vi "main_original.vi"() -> ()   [LabVIEW 2010]
uses:
  common_typedefs/channels_cluster.ctl
  common_typedefs/clock_parameters_cluster.ctl
  scan_specification_cluster.ctl
  common_typedefs/DAC_voltage_cluster.ctl
  derived_values_cluster.ctl
  counter_cluster.ctl
  integration_cluster.ctl
  common_typedefs/DAC_values_cluster.ctl
  common_typedefs/DAC_channel_enable_cluster.ctl
  <vilib>/Platform/TimedLoop/XDataNode/XDataNode.xnode
  <vilib>/Platform/TimedLoop/XDataNode/timing_clust.ctl
  <vilib>/Platform/TimedLoop/XDataNode/nitl_modes.ctl
  <vilib>/Platform/TimedLoop/XDataNode/wakeup.ctl
  <vilib>/eio/EIONode/EIONode.xnode
  <vilib>/rvi/eio/nirviEIOImplementation/nirviEIOImplementation.xnode
  <vilib>/rvi/eio/common/nirviEmuClasses.ctl
  <vilib>/rvi/eio/common/nirviEmuTemplateMethod_noerrors.vi
  <vilib>/Platform/TimedLoop/XDataNode/XDNodeRunTimeDep.lvlib
panel:
  in  "sync minimum high":i16=1000
  out "PIXEL COUNTER":u64(graph)
  out "Loop time":u32=100
  out "line counter":u16(graph)
  out "finished?":bool
  in  "transfer extra-waitlines?":bool
  out "transferred extra waitlines":u32
  out "no of correct transferred z tuples":u32
  out "z-points transfer corrupt?":bool
  out "transferred z/intensity tuples":u32
  in  "transfer z-points?":bool
  in  "invert channels":bool[](array[boolean])=[FALSE, FALSE]
  in  "enable fly-back reversion?":bool=TRUE
  out "pixels acquired":u64
  out "counter cluster out":T1
  out "derived values":T2
  out "acquire?":bool
  in  "ADC clock phase":u8=2
  out "DAC voltages":T3 {"ch6" max=4095 step=1; "ch5" max=4095 step=1; "ch4" max=4095 step=1; "ch3" max=4095 step=1; "ch2" max=4095 step=1; "ch1" max=4095 step=1; "ch0" max=4095 step=1}
  in  "scan specification":T4={"x amplitude"=1000, "x resolution (pixels)"=100, "x offset fly-forward (iterations)"=0, "x offset fly-back (iterations)"=0, "y resolution (nr. of lines)"=200, "y step size"=5, "iterations per pixel"=5, "number of frames"=-1, "y offset (pixels)"=0, "number of y-brake lines  (before y-fly-back)"=2, "number y-brake lines (after y-fly-back)"=2, "number of y-fly-back steps"=2, "lines per z step"=5, "number of z/intensity tuples"=200, "number of repetitions (volumes or planes)"=500, "z step size derived"=0, "choose the beginning of z scan"=FALSE, "number of frames (settings)"=0, "FPGA trajectory?"=FALSE}
  out "clock 1 state":bool
  out "clock 2 state":bool
  out "clock 3 state":bool
  in  "clock 2 settings":T5
  in  "clock 1 settings":T5
  in  "clock 3 settings":T5
  out "data read":T6
  in  "maximum bit depth":i8
  out "FIFO overflow":bool
  in  "scan":bool
  in  "stop":bool
  in  "wait for trigger?":bool
  in  "stop acquisition at\nFIFO overflow?":bool
  out "scanning?":bool
  in  "converter box version":i16=2 min=1 max=2
  # "Mirna: \niterations per pixel = (x scan segment fraction*fFPGA)/(x resolution*f resonance)\nfFPGA/f resonance = 5000 --assumes 8kHz resonance frequency\niterations per pixel=25"
  # "used to be 1000 (Mirna)"
  # "y settings:\ny resolution*y step size = 6553\nthis gives scan from -1 to 1V\ny resolution = 200\ny step size = 33\n\nz settings:\nto scan entire y profile \nnumber of z's has to be equal\ny resolution"
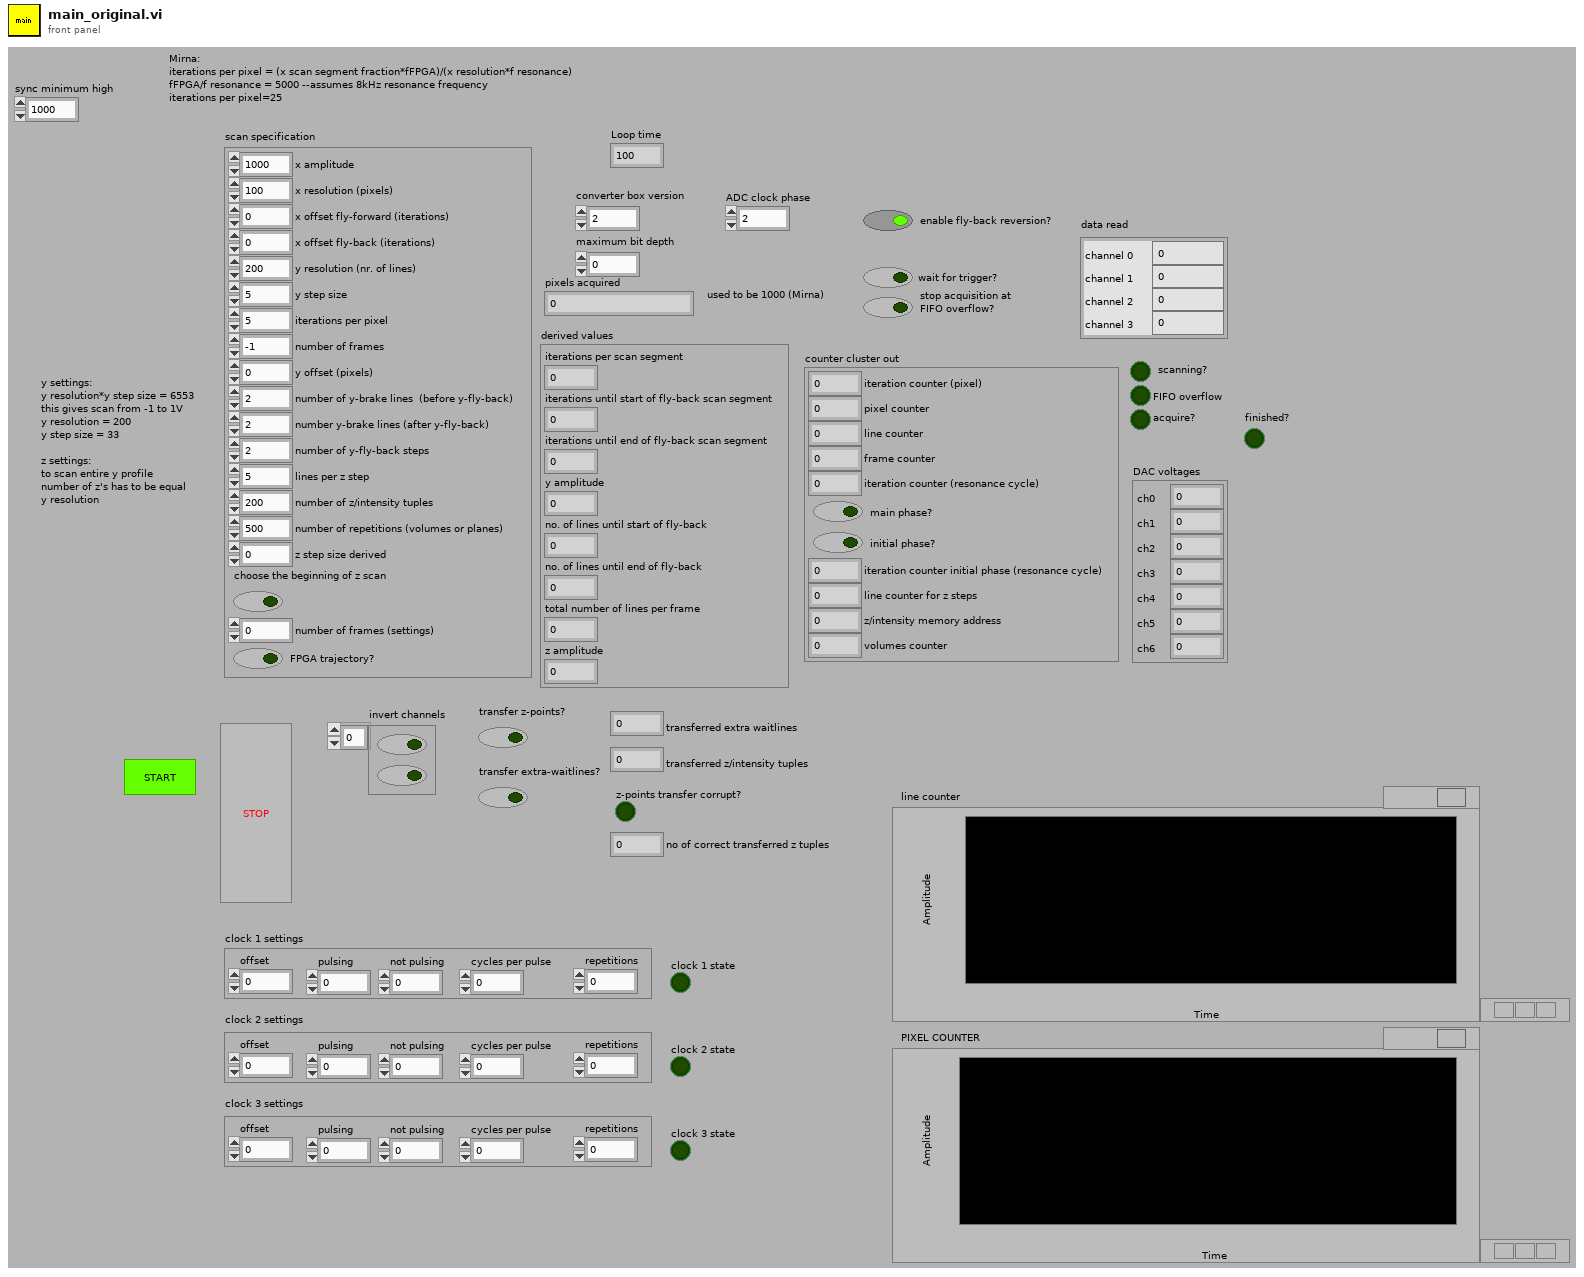
[diagram p1: front panel]
types:
  T1 = typedef "counter_cluster.ctl" = cluster{"iteration counter (pixel)":u16, "pixel counter":u16, "line counter":u16, "frame counter":u16, "iteration counter (resonance cycle)":u16, "main phase?":bool, "initial phase?":bool, "iteration counter initial phase (resonance cycle)":u16, "line counter for z steps":u16, "z/intensity memory address":u32, "volumes counter":u16}
  T2 = typedef "derived_values_cluster.ctl" = cluster{"iterations per scan segment":u16, "iterations until start of fly-back scan segment":u16, "iterations until end of fly-back scan segment":u16, "y amplitude":u16, "no. of lines until start of fly-back":u16, "no. of lines until end of fly-back":u16, "total number of lines per frame ":u16, "z amplitude":u16}
  T3 = typedef "DAC_voltage_cluster.ctl" = cluster{"ch0":u16, "ch1":i16, "ch2":i16, "ch3":u16, "ch4":u16, "ch5":u16, "ch6":u16}
  T4 = typedef "scan_specification_cluster.ctl" = cluster{"x amplitude":u16, "x resolution (pixels)":u16, "x offset fly-forward (iterations)":u16, "x offset fly-back (iterations)":u16, "y resolution (nr. of lines)":u16, "y step size":u16, "iterations per pixel":u16, "number of frames":i32, "y offset (pixels)":u16, "number of y-brake lines  (before y-fly-back)":u16, "number y-brake lines (after y-fly-back)":u16, "number of y-fly-back steps":u16, "lines per z step":u16, "number of z/intensity tuples":u16, "number of repetitions (volumes or planes)":i32, "z step size derived":u16, "choose the beginning of z scan":bool, "number of frames (settings)":i32, "FPGA trajectory?":bool}
  T5 = typedef "clock_parameters_cluster.ctl" = cluster{"offset":i64, "pulsing":i64, "not pulsing":i64, "cycles per pulse":i64, "repetitions":i64}
  T6 = typedef "channels_cluster.ctl" = cluster{"channel 0":u32, "channel 1":u32, "channel 2":u32, "channel 3":u32}
  T7 = typedef "DAC_values_cluster.ctl" = cluster{"DAC channel enable":T8, "DAC voltage":T3, "offset":u16, "channel index":u16, "bit index":i32, "synch?":bool, "DAC clock":bool, "finished?":bool}
  T8 = typedef "DAC_channel_enable_cluster.ctl" = cluster{"ch0":bool, "ch1":bool, "ch2":bool, "ch3":bool, "ch4":bool, "ch5":bool, "ch6":bool}
  T9 = typedef "integration_cluster.ctl" = cluster{"channel 0":u32, "channel 1":u32, "fly-back heap address":u32}
  T10 = typedef "XDNodeRunTimeDep.lvlib/timing_clust.ctl" = cluster{"Expected End [f-1]":u64, "Actual End [f-1]":u64, "Finished Late? [f-1]":bool, "Expected End [i-1]":u64, "Actual End [i-1]":u64, "Finished Late? [i-1]":bool, "Expected Start [i]":u64, "Actual Start [i]":u64, "Expected Start [f]":u64, "Actual Start [f]":u64, "Source Name":string, "Structure Name":string, "Period":i64, "Deadline":i64, "Offset":i64, "Start":i64, "Priority":i32, "Timeout":i32, "Mode":T11, "Wakeup Reason":T12, "Error":errorcluster, "Source Type":string, "Secondary Source Type":string, "Global End Time":u64, "Global Start Time":u64, "Frame Duration":u64, "Iteration Duration":u64, "Assigned CPU":i32, "I/O Scan Engine Mode":u32}
  T11 = typedef "XDNodeRunTimeDep.lvlib/nitl_modes.ctl" = enum32{"No Change", "Process missed periods, maintain original phase", "Discard missed periods, maintain original phase", "Process missed periods, ignore original phase", "Discard missed periods, ignore original phase"}
  T12 = typedef "XDNodeRunTimeDep.lvlib/wakeup.ctl" = enum32{"Normal", "Aborted", "Asynchronous wakeup", "Timing source error", "Timed loop error", "Timeout"}
  T13 = typedef "nirviEmuClasses.ctl" = enum16{"IO Read", "IO Write", "Method", "Property Read", "Property Write"}
  T14 = typedef "gate_counters_cluster.ctl" = cluster{"phase iteration counter":i64, "phase repetition counter":i64, "pulse iteration counter":i64, "phase state":bool}
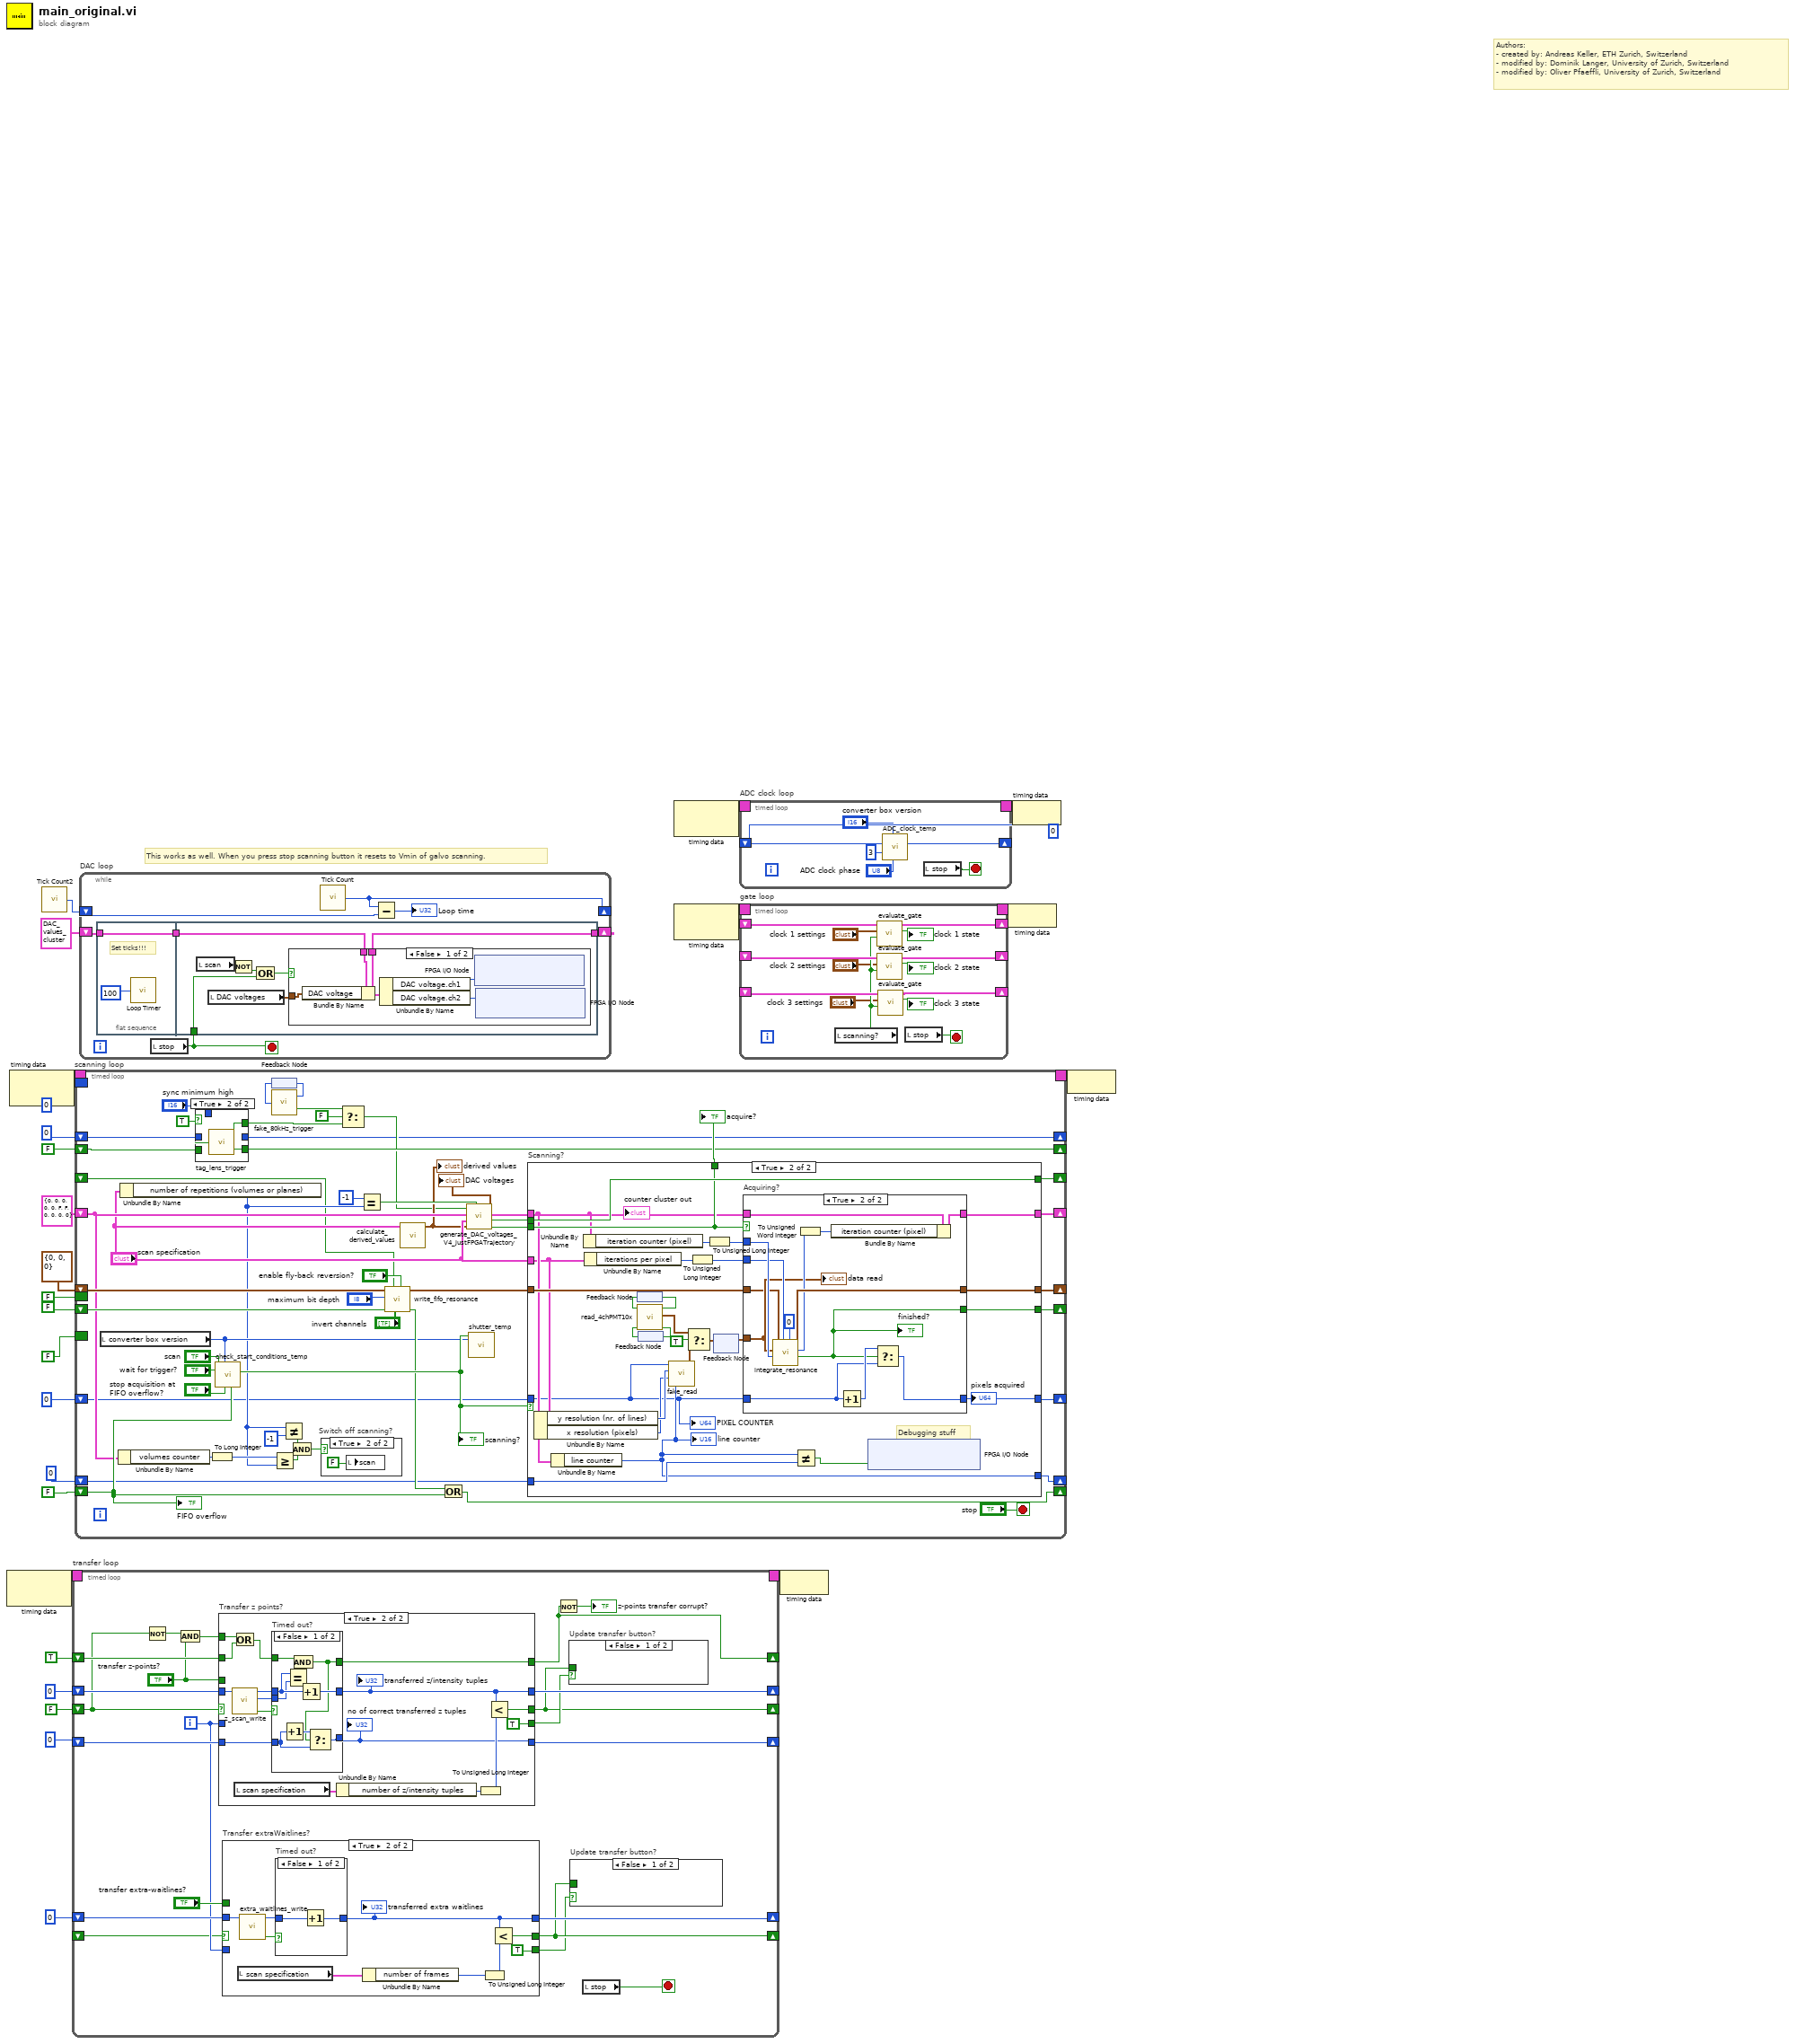
[diagram p0: block diagram]
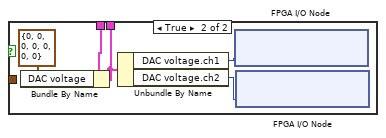
[diagram p2: hidden frame]
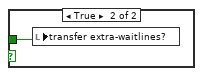
[diagram p3: hidden frame]
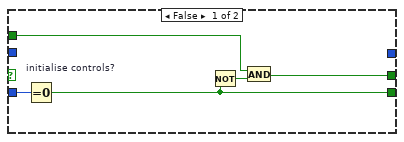
[diagram p4: hidden frame]
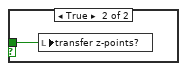
[diagram p6: hidden frame]
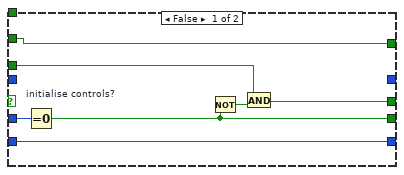
[diagram p7: hidden frame]
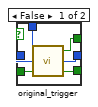
[diagram p9: hidden frame]
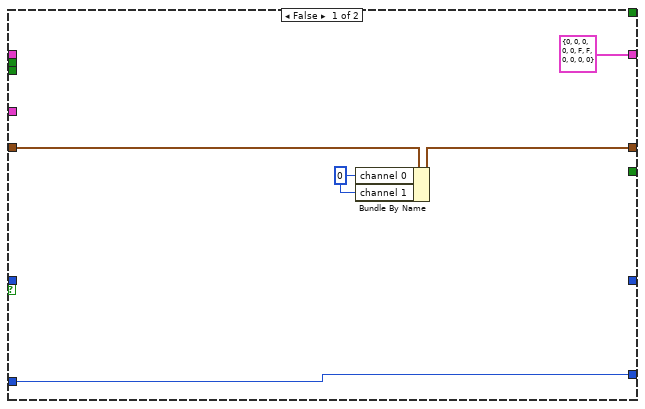
[diagram p11: hidden frame]
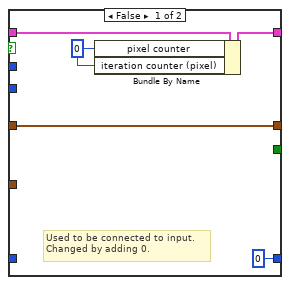
[diagram p12: hidden frame]
diagram:
  # "This works as well. When you press stop scanning button it resets to Vmin of galvo scanning."
  # "Authors: \n- created by: Andreas Keller, ETH Zurich, Switzerland\n- modified by: Dominik Langer, University of Zurich, Switzerland\n- modified by: Oliver Pfaeffli, University of Zurich, Switzerland"
  n1 = node-c288() -> (w12:T10)  [unwired: 1 in]
  n2 = node-c288() -> (w25:T10)  [unwired: 1 in]
  n3 = call "Tick Count2"() -> ("Tick Count(Ticks)"=w5:u32)
  n4 = timed-loop "transfer loop" {
    shift-right: [w47] -> _
    shift-left: u32 0 ("address out") -> [w48]
    timing: w12 -> [_]
    timing-out: [_] -> w11
    shift-right: [w45] -> _
    shift-left: FALSE ("start z-points transfer?") -> [w40]
    shift-right: [w43] -> _
    shift-left: TRUE ("start z-points transfer?") -> [w44]
    shift-right: [w36] -> _
    shift-left: u32 0 ("address out") -> [w37]
    shift-right: [w34] -> _
    shift-left: u32 0 ("address extra waitlines OUT") -> [w35]
    shift-right: [w30] -> _
    shift-left: _ -> [w31]
    i -> [w32]
    stop <- w28 stop-if-true
    n5 = Not(x=w40) -> (.not. x?=w41:bool)
    n6 = And(x=w41, y="transfer z-points?") -> (x .and. y?=w38:bool)
    n7 = case "Transfer z points?" shown="True" w40 {
      tunnel: w48 -> [_ w90]
      tunnel: [_ w88] -> w47
      tunnel: [w72 w84] -> w45
      tunnel: w32 -> [w74 _]
      tunnel: [w71 TRUE] -> w46
      tunnel: w44 -> [w70 w78]
      tunnel: [w70 w80] -> w43
      tunnel: "transfer z-points?" -> [w69 _]
      tunnel: w38 -> [_ w79]
      tunnel: w37 -> [w68 w76]
      tunnel: [w68 w75] -> w36
      frame False {
        n8 = Equal To 0? "initialise controls?"(x=w74) -> (x = 0?=w71:bool)
        n9 = Not(x=w71) -> (.not. x?=w73:bool)
        n10 = And(x=w69, y=w73) -> (x .and. y?=w72:bool)
      }
      frame True {
        n11 = Or(x=w79, y=w78) -> (x .or. y?=w77:bool)
        n12 = call "z_scan_write.vi"("address in"=w90) -> ("FIFO scan time out"=w82:bool, "data"=w81:u32, "address out"=w89:u32)  [unwired: 8 in]
        n13 = local read "scan specification"() -> (w87:T4)
        n14 = case "Timed out?" shown="False" w82 {
          tunnel: w89 -> [w96 w102]
          tunnel: [w99 w102] -> w88
          tunnel: w81 -> [w95 _]
          tunnel: w77 -> [w98 w101]
          tunnel: [w92 w101] -> w80
          tunnel: w76 -> [w94 w100]
          tunnel: [w91 w100] -> w75
          frame False {
            n15 = Increment(x=w94) -> (x+1=w93:u32)
            n16 = Equal?(x=w96, y=w95) -> (x = y?=w97:bool)
            n17 = And(x=w98, y=w97) -> (x .and. y?=w92:bool)
            n18 = Increment(x=w96) -> (x+1=w99:u32)
            n19 = Select(t=w93, s=w92, f=w94) -> (s? t:f=w91:u32)
          }
          frame True {
          }
        }
        "transferred z/intensity tuples" <- w88
        "no of correct transferred z tuples" <- w75
        n20 = Unbundle By Name(w87) -> ("number of z/intensity tuples"=w86:u16)
        n21 = To Unsigned Long Integer(number=w86) -> (unsigned 32bit integer=w85:u32)
        n22 = Less?(x=w88, y=w85) -> (x < y?=w84:bool)
      }
    }
    n23 = case "Transfer extraWaitlines?" shown="True" w31 {
      tunnel: [_ w63] -> w34
      tunnel: [w53 w60] -> w30
      tunnel: [w52 TRUE] -> w29
      tunnel: w35 -> [_ w56]
      tunnel: "transfer extra-waitlines?" -> [w50 _]
      tunnel: w32 -> [w51 _]
      frame False {
        n24 = Equal To 0? "initialise controls?"(x=w51) -> (x = 0?=w52:bool)
        n25 = Not(x=w52) -> (.not. x?=w54:bool)
        n26 = And(x=w50, y=w54) -> (x .and. y?=w53:bool)
      }
      frame True {
        n27 = local read "scan specification"() -> (w58:T4)
        n28 = call "extra_waitlines_write.vi"("address extra waitlines IN"=w56) -> ("FIFO scan time out"=w55:bool, "address extra waitlines OUT"=w57:u32)  [unwired: 8 in, 1 out]
        n29 = case "Timed out?" shown="False" w55 {
          tunnel: w57 -> [w64 w66]
          tunnel: [w65 w66] -> w63
          frame False {
            n30 = Increment(x=w64) -> (x+1=w65:u32)
          }
          frame True {
          }
        }
        "transferred extra waitlines" <- w63
        n31 = Unbundle By Name(w58) -> ("number of frames"=w62:i32)
        n32 = To Unsigned Long Integer(number=w62) -> (unsigned 32bit integer=w61:u32)
        n33 = Less?(x=w63, y=w61) -> (x < y?=w60:bool)
      }
    }
    n34 = Not(x=w43) -> (.not. x?=→"z-points transfer corrupt?":bool)
    n35 = case "Update transfer button?" shown="False" w46 {
      tunnel: w45 -> [_ w67]
      frame False {
      }
      frame True {
        n36 = local write "transfer z-points?"(w67) -> ()
      }
    }
    n37 = case "Update transfer button?" shown="False" w29 {
      tunnel: w30 -> [_ w49]
      frame False {
      }
      frame True {
        n38 = local write "transfer extra-waitlines?"(w49) -> ()
      }
    }
    n39 = local read "stop"() -> (w28:bool)
  }
  n40 = timed-loop "scanning loop" {
    timing: w25 -> [_]
    timing-out: [_] -> w24
    shift-right: [w155] -> _
    shift-left: T1 {"iteration counter (pixel)"=0, "pixel counter"=0, "line counter"=0, "frame counter"=0, "iteration counter (resonance cycle)"=0, "main phase?"=FALSE, "initial phase?"=FALSE, "iteration counter initial phase (resonance cycle)"=0, "line counter for z steps"=0, "z/intensity memory address"=0, "volumes counter"=0} ("counter cluster") -> [w134]
    shift-right: [w142] -> _
    shift-left: T9 {"channel 0"=0, "channel 1"=0, "fly-back heap address"=0} ("integration cluster") -> [w141]
    shift-right: [w144] -> _
    shift-left: FALSE -> [w136]
    shift-right: [w148] -> _
    shift-left: u64 0 -> [w106]
    shift-right: [w109] -> _
    shift-left: i16 0 -> [w110]
    shift-right: [w143] -> _
    shift-left: _ -> [w107]
    shift-right: [w138] -> _
    shift-left: FALSE ("finished?") -> [w137]
    shift-right: [w115] -> _
    shift-left: FALSE -> [w116]
    shift-right: [w119] -> _
    shift-left: u64 0 -> [w120]
    border: FALSE ("Inputl1") -> [_]
    border: FALSE ("Input0") -> [_]
    border: u16 0 -> [_]
    stop <- "stop" stop-if-true
    n41 = local read "converter box version"() -> (w126:i16)
    n42 = Unbundle By Name(w134) -> ("volumes counter"=w130:u16)
    n43 = Unbundle By Name("scan specification") -> ("number of repetitions (volumes or planes)"=w124:i32)
    n44 = case shown="True" TRUE {
      tunnel: w116 -> [w159 w164]
      tunnel: [w161 w166] -> w111
      tunnel: [w160 w165] -> w115
      tunnel: w110 -> [w163 _]
      tunnel: [w162 _] -> w109
      tunnel: "sync minimum high" -> [w158 _]
      frame False {
        n45 = call "original_trigger.vi"("last sync value"=w159, "counter in"=w163, "sync minimum high"=w158) -> ("DIO stored in shift registar"=w160:bool, "counter out"=w162:i16, "trigger out"=w161:bool)
      }
      frame True {
        n46 = call "tag_lens_trigger.vi"("previous DIO value"=w164) -> ("DIO to shift registar"=w165:bool, "trigger out"=w166:bool)
      }
    }
    n47 = To Long Integer(number=w130) -> (32bit integer=w129:i32)
    n48 = call "check_start_conditions_temp.vi"("FIFO overflow?"=w136, "stop at FIFO overflow?"="stop acquisition at\nFIFO overflow?", "converter box version"=w126, "in triggered mode?"="wait for trigger?", "acquire"="scan") -> ("acquire?"=w150:bool)  [unwired: 6 in]
    "scanning?" <- w150
    n49 = feedback #1() -> (w125:u16)
    n50 = call "fake_80kHz_trigger.vi"("Counter in"=w125) -> ("trigger"=w112:bool, "Counter out"=w121:u16)
    n51 = feedback-in #1(w121) -> ()
    n52 = Greater Or Equal?(x=w129, y=w124) -> (x >= y?=w152:bool)
    n53 = Not Equal?(x=w124, y=-1) -> (x != y?=w149:bool)
    n54 = And(x=w149, y=w152) -> (x .and. y?=w122:bool)
    n55 = case "Switch off scanning?" shown="True" w122 {
      frame False {
      }
      frame True {
        n56 = local write "scan"(FALSE ("scan")) -> ()
      }
    }
    n57 = Select(t=w112, s=FALSE, f=w111) -> (s? t:f=w114:bool)
    n58 = Equal?(x=-1, y=w124) -> (x = y?=w127:bool)
    n59 = call "write_fifo_resonance.vi"("enable fly-back reversion?"="enable fly-back reversion?", "invert channels"="invert channels", "fly-back?"=w107, "pixel finished?"=w137, "maximum bit depth"="maximum bit depth", "integration cluster in"=w141) -> ("FIFO overflow out"=w139:bool, "integration cluster out"=w140:T9)  [unwired: 4 in]
    n60 = call "calculate_derived_values.vi"("scan specification"="scan specification") -> ("derived values"=w123:T2)  [unwired: 10 in]
    "derived values" <- w123
    n61 = Or(x=w139, y=w136) -> (x .or. y?=w144:bool)
    n62 = call "generate_DAC_voltages_V4_justFPGATrajectory.vi"("focus mode?"=w127, "derived values"=w123, "scan specification"="scan specification", "counter cluster in"=w134, "resonant trigger"=w114) -> ("acquire?"=w131:bool, "fly-back acquisition phase?"=w105:bool, "counter cluster out"=w133:T1, "DAC voltages"=→"DAC voltages":T3)  [unwired: 3 in]
    n63 = call "shutter_temp.vi"("converter box version"=w126, "open?"=w150) -> ()  [unwired: 10 in]
    n64 = case "Scanning?" shown="True" w150 {
      tunnel: w133 -> [_ w189]
      tunnel: [T1 {"iteration counter (pixel)"=0, "pixel counter"=0, "line counter"=0, "frame counter"=0, "iteration counter (resonance cycle)"=0, "main phase?"=FALSE, "initial phase?"=FALSE, "iteration counter initial phase (resonance cycle)"=0, "line counter for z steps"=0, "z/intensity memory address"=0, "volumes counter"=0} ("counter cluster") w200] -> w155
      tunnel: w140 -> [w170 w196]
      tunnel: [w169 w199] -> w142
      tunnel: "scan specification" -> [_ w181]
      tunnel: w106 -> [_ w173]
      tunnel: [_ w193] -> w148
      tunnel: [_ w190] -> w147
      tunnel: [_ w192] -> w138
      tunnel: [_ w191] -> w143
      tunnel: w105 -> [_ w191]
      tunnel: w131 -> [_ w190]
      tunnel: [w168 w176] -> w119
      tunnel: w120 -> [w168 w188]
      frame False {
        w171 = u32 0 ("channel 0")
        n65 = Bundle By Name(cluster=w170, "channel 0"=w171, "channel 1"=w171) -> (w169:T9)
      }
      frame True {
        # "Debugging stuff"
        n66 = Unbundle By Name(w181) -> ("y resolution (nr. of lines)"=w175:u16, "x resolution (pixels)"=w174:u16)
        n67 = Unbundle By Name(w189) -> ("line counter"=w176:u16)
        "line counter" <- w176
        n68 = Unbundle By Name(w189) -> ("iteration counter (pixel)"=w198:u16)
        n69 = Unbundle By Name(w181) -> ("iterations per pixel"=w197:u16)
        n70 = feedback #2() -> (w183:bool)
        n71 = feedback #3() -> (w185:bool)
        n72 = call "read_4chPMT10x.vi"("previous value ch1"=w185, "previous value ch0"=w183) -> ("Inputl1"=w184:bool, "read output"=w180:T6, "Input0"=w186:bool)  [unwired: 7 in]
        n73 = feedback-in #2(w186) -> ()
        n74 = feedback-in #3(w184) -> ()
        n75 = call "fake_read.vi"("line counter"=w176, "x resolution (pixels)"=w174, "y resolution (nr. of lines)"=w175, "Numeric"=w173) -> ("input cluster"=w177:T6)
        n76 = Select(t=w180, s=TRUE, f=w177) -> (s? t:f=w179:T6)
        n77 = To Unsigned Long Integer(number=w197) -> (unsigned 32bit integer=w194:u32)
        n78 = To Unsigned Long Integer(number=w198) -> (unsigned 32bit integer=w195:u32)
        n79 = feedback #4() -> (w182:T6)  [unwired: 1 in]
        n80 = feedback-in #4(w179) -> ()
        n81 = case "Acquiring?" shown="True" w190 {
          tunnel: w189 -> [w215 w225]
          tunnel: [w216 w223] -> w200
          tunnel: [w213 w228] -> w199
          tunnel: w196 -> [w213 w221]
          tunnel: w195 -> [_ w229]
          tunnel: w182 -> [_ w224]
          tunnel: w194 -> [_ w226]
          tunnel: w173 -> [_ w218]
          tunnel: [u64 0 w220] -> w193
          tunnel: [_ w217] -> w192
          frame False {
            w214 = u16 0 ("pixel counter")
            # "Used to be connected to input.\nChanged by adding 0."
            n82 = Bundle By Name(cluster=w215, "pixel counter"=w214, "iteration counter (pixel)"=w214) -> (w216:T1)
          }
          frame True {
            n83 = call "integrate_resonance.vi"("waiting iterations per pixel"=u32 0, "integration iterations per pixel"=w226, "iteration counter in"=w229, "sampling values in"=w224, "integration cluster in"=w221) -> ("finished?"=w217:bool, "iteration counter out"=w227:u32, "integration cluster out"=w228:T9)  [unwired: 4 in]
            "finished?" <- w217
            n84 = To Unsigned Word Integer(number=w227) -> (unsigned 16bit integer=w230:u16)
            n85 = Bundle By Name(cluster=w225, "iteration counter (pixel)"=w230) -> (w223:T1)
            n86 = Increment(x=w218) -> (x+1=w219:u64)
            n87 = Select(t=w219, s=w217, f=w218) -> (s? t:f=w220:u64)
            "data read" <- w224
          }
        }
        "pixels acquired" <- w193
        n88 = Not Equal?(x=w176, y=w188) -> (x != y?=w187:bool)
        n89 = xnode "FPGA I/O Node"("Connector0/DIO0"=w187) -> ()  [unwired: 1 in, 1 out]
        "counter cluster out" <- w189
        "PIXEL COUNTER" <- w173
      }
    }
    "acquire?" <- w147
    "FIFO overflow" <- w136
  }
  n90 = while "DAC loop" {
    shift-right: [w239] -> _
    shift-left: T7 {"DAC channel enable"={"ch0"=FALSE, "ch1"=FALSE, "ch2"=FALSE, "ch3"=FALSE, "ch4"=FALSE, "ch5"=FALSE, "ch6"=FALSE}, "DAC voltage"={"ch0"=0, "ch1"=0, "ch2"=0, "ch3"=0, "ch4"=0, "ch5"=0, "ch6"=0}, "offset"=0, "channel index"=0, "bit index"=0, "synch?"=FALSE, "DAC clock"=FALSE, "finished?"=FALSE} ("DAQ values out") -> [w238]
    shift-right: [w236] -> _
    shift-left: w5 -> [w235]
    stop <- w233 stop-if-true
    n91 = flat-sequence {
      tunnel: w238 -> [w241]
      tunnel: [w241] -> w237
      tunnel: [w248] -> w239
      tunnel: w237 -> [w247]
      tunnel: w233 -> [w246]
      frame #0 {
        # "Set ticks!!!"
        n92 = call "Loop Timer"("Count(Ticks)"=u32 100) -> ()  [unwired: 1 out]
      }
      frame #1 {
        n93 = local read "scan"() -> (w243:bool)
        n94 = local read "DAC voltages"() -> (w242:T3)
        n95 = Not(x=w243) -> (.not. x?=w244:bool)
        n96 = Or(x=w244, y=w246) -> (x .or. y?=w245:bool)
        n97 = case shown="False" w245 {
          tunnel: w242 -> [w251 _]
          tunnel: w247 -> [w250 w279]
          tunnel: [w249 w276] -> w248
          frame False {
            n98 = Bundle By Name(cluster=w250, "DAC voltage"=w251) -> (w249:T7)
            n99 = Unbundle By Name(w249) -> ("DAC voltage.ch1"=w252:i16, "DAC voltage.ch2"=w253:i16)
            n100 = xnode "FPGA I/O Node"("Connector0/AO0"=w252) -> ()  [unwired: 1 in, 1 out]
            n101 = xnode "FPGA I/O Node"("Connector0/AO1"=w253) -> ()  [unwired: 1 in, 1 out]
          }
          frame True {
            n102 = Bundle By Name(cluster=w279, "DAC voltage"=T3 {"ch0"=0, "ch1"=0, "ch2"=0, "ch3"=0, "ch4"=0, "ch5"=0, "ch6"=0}) -> (w276:T7)
            n103 = Unbundle By Name(w276) -> ("DAC voltage.ch1"=w277:i16, "DAC voltage.ch2"=w278:i16)
            n104 = xnode "FPGA I/O Node"("Connector0/AO0"=w277) -> ()  [unwired: 1 in, 1 out]
            n105 = xnode "FPGA I/O Node"("Connector0/AO1"=w278) -> ()  [unwired: 1 in, 1 out]
          }
        }
      }
    }
    n106 = local read "stop"() -> (w233:bool)
    n107 = call "Tick Count"() -> ("Tick Count(Ticks)"=w236:u32)
    n108 = Subtract(x=w236, y=w235) -> (x-y=→"Loop time":u32)
  }
  n109 = node-c288() -> (w16:T10)  [unwired: 1 out]
  n110 = node-c288() -> (w27:T10)  [unwired: 1 in]
  n111 = timed-loop "ADC clock loop" {
    timing: w16 -> [_]
    timing-out: [_] -> w15
    shift-right: [w305] -> _
    shift-left: u8 0 -> [w306]
    stop <- w308 stop-if-true
    n112 = call "ADC_clock_temp.vi"("phase"="ADC clock phase", "converter box version"="converter box version", "iterations per cycle"=u8 3, "counter in"=w306) -> ("counter out"=w305:u8)  [unwired: 7 in]
    n113 = local read "stop"() -> (w308:bool)
  }
  n114 = timed-loop "gate loop" {
    timing: w27 -> [_]
    timing-out: [_] -> w26
    shift-right: [w323] -> _
    shift-left: _ -> [w324]
    shift-right: [w320] -> _
    shift-left: _ -> [w319]
    shift-right: [w321] -> _
    shift-left: _ -> [w318]
    stop <- w322 stop-if-true
    n115 = local read "scanning?"() -> (w317:bool)
    n116 = call "evaluate_gate.vi"("acquiring?"=w317, "gate settings"="clock 1 settings", "gate counters in"=w324) -> ("pulse state out"=→"clock 1 state":bool, "gate counters out"=w323:T14)  [unwired: 7 in]
    n117 = call "evaluate_gate.vi"("acquiring?"=w317, "gate settings"="clock 2 settings", "gate counters in"=w319) -> ("pulse state out"=→"clock 2 state":bool, "gate counters out"=w320:T14)  [unwired: 7 in]
    n118 = call "evaluate_gate.vi"("acquiring?"=w317, "gate settings"="clock 3 settings", "gate counters in"=w318) -> ("pulse state out"=→"clock 3 state":bool, "gate counters out"=w321:T14)  [unwired: 7 in]
    n119 = local read "stop"() -> (w322:bool)
  }
  n120 = node-c288(w11) -> ()
  n121 = node-c288(w26) -> ()
  n122 = node-c288(w15) -> ()
  n123 = node-c288(w24) -> ()
